vi "LM model function_1 width.vi"(3 "output control":T1, 4 "data":variant, 5 "X":dbl[](array[numeric]), 6 "a":dbl[](array[numeric])) -> (0 "error out":errorcluster, 1 "f'(X,a)":dbl[][](array[numeric]), 2 "f(X,a)":dbl[](array[numeric]))   [LabVIEW 2016]
doc: "This template is the starting point for creating a model function to be passed to the Nonlinear Curve Fit.vi."
uses:
  <vilib>/gmath/NumericalOptimization/LM_output select.ctl
  <vilib>/gmath/NI_Gmath.lvlib
panel:
  out "loop":i32
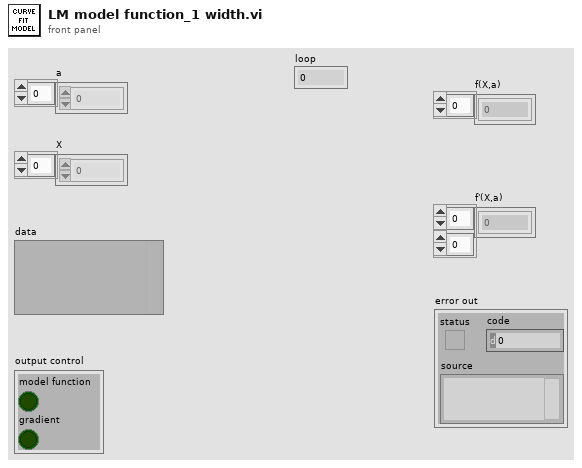
[diagram p1: front panel]
types:
  T1 = typedef "NI_Gmath.lvlib/LM_output select.ctl" = cluster{"model function":bool, "gradient":bool}
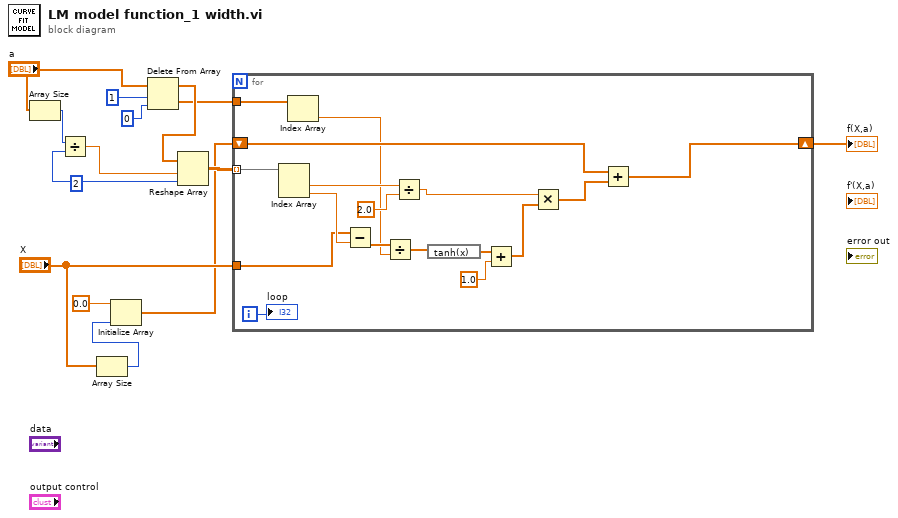
[diagram p0: block diagram]
diagram:
  w7 = 2 ("dimension size")
  n1 = Array Size(array="a") -> (size(s)=w8:i32)
  n2 = Divide(x=w8, y=w7) -> (x/y=w6:dbl)
  n3 = Array Size(array="X") -> (size(s)=w11:i32)
  n4 = Initialize Array(0.0 ("element"), w11) -> (w10:dbl[])
  n5 = Delete From Array(array="a", length=1, index=0) -> (deleted portion=w1:dbl[], array with subset deleted=w2:dbl[])
  n6 = Reshape Array(w2, w6, w7) -> (w14:dbl[][])
  n7 = for {
    tunnel: w14 -> [w31] mode=indexing
    tunnel: "X" -> [w18]
    shift-right: [w20] -> w9
    shift-left: w10 -> [w21]
    tunnel: w1 -> [w16]
    i -> [w17]
    n8 = Index Array(array=w31) -> (element #1=w30:dbl, element #2=w19:dbl)  [unwired: 2 in]
    n9 = Index Array(array=w16) -> (element=w15:dbl)  [unwired: 1 in]
    n10 = Subtract(x=w18, y=w19) -> (x-y=w27:dbl[])
    n11 = Divide(x=w27, y=w15) -> (x/y=w26:dbl[])
    n12 = Divide(x=w30, y=2.0) -> (x/y=w28:dbl)
    n13 = expression code="tanh(x)"(w26) -> (w25:dbl[])
    n14 = Add(x=w25, y=1.0) -> (x+y=w23:dbl[])
    n15 = Multiply(x=w28, y=w23) -> (x*y=w22:dbl[])
    n16 = Add(x=w21, y=w22) -> (x+y=w20:dbl[])
    "loop" <- w17
  }
  "f(X,a)" <- w9
